vi "subOpenAppBuilderVI.vi"(11 "Application in":refnum<vi>) -> (3 "VI ref":refnum<vi>)   [LabVIEW 2020, in "SolutionBuilder.lvlib" / "SolutionBuilder.lvclass"]
uses:
  SolutionBuilder.lvclass
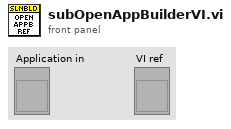
[diagram p1: front panel]
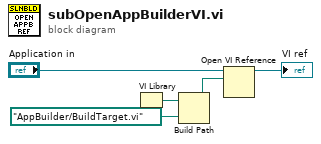
[diagram p0: block diagram]
diagram:
  n1 = VI Library() -> (path=w2:path)
  n2 = Build Path(base path=w2, name or relative path=path "AppBuilder/BuildTarget.vi" ("vi path")) -> (appended path=w4:path)
  n3 = Open VI Reference(application reference (local)="Application in", vi path=w4) -> (vi reference=→"VI ref":refnum<vi>)  [unwired: 2 in, 3 out]
